vi "JIG_RESET_encode.vi"(8 "error in (no error)":errorcluster, 10 "JIG RESET":bool, 11 "Mem_mapping in":u16[](array[numeric])) -> (0 "error out":errorcluster, 3 "MemMapping Out":u16[](array[numeric]))   [LabVIEW 2018, in "MB Relay.lvlib"]
uses:
  MB Relay.lvlib
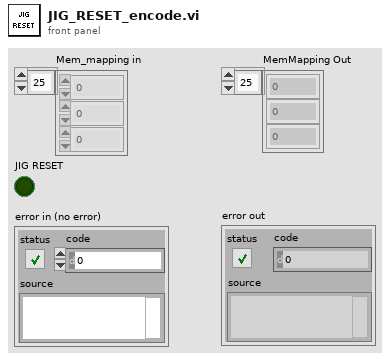
[diagram p1: front panel]
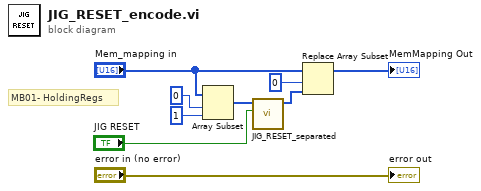
[diagram p0: block diagram]
diagram:
  # "MB01- HoldingRegs"
  n1 = Array Subset(array="Mem_mapping in", index=0, length=1) -> (w3:u16[])
  n2 = call "JIG_RESET_separated.vi"("JIG_RESET"="JIG RESET", "Mem_mapping in"=w3) -> ("Mem_mapping out"=w1:u16[])  [unwired: 9 in]
  n3 = Replace Array Subset(array="Mem_mapping in", new element=w1, index=0) -> (→"MemMapping Out":u16[])
  "error out" <- "error in (no error)"
